vi "Begin.vi"(11 "Image Size":T3=enum."160x120") -> (0 "error out":errorcluster)   [LabVIEW 2011]
doc: "Called before other user functions, this VI is expected to open initial I/O refnums, load in file data, and do all program initialization. Notice that the <B>error out</B> terminal is simply used for data flow. Wiring it to other structures or subVIs ensures that this VI runs first."
uses:
  <vilib>/Rock Robotics/WPI/Camera/WPI_CameraImageSize.ctl
  <vilib>/Rock Robotics/SystemInterfaces/AI/FPGA_AIGyroChannel.ctl
  <vilib>/Rock Robotics/SystemInterfaces/Typedef/FPGA_TypedefAnalogModuleForGyro.ctl
  <vilib>/Rock Robotics/WPI/Joystick/WPI_JoystickDeviceEnum.ctl
  <vilib>/Rock Robotics/WPI/Camera/WPI_CameraWhite Balance Values.ctl
  <vilib>/Rock Robotics/WPI/Camera/WPI_CameraExposure Values.ctl
  <vilib>/Rock Robotics/WPI/Camera/WPI_CameraFrameRate.ctl
  <vilib>/Rock Robotics/WPI/CAN/Jaguar/SubVIs/WPI_CANJaguar_BrakeCoastMode.ctl
  <vilib>/Rock Robotics/WPI/CAN/Jaguar/SubVIs/WPI_CANJaguar_ControlMode.ctl
  <vilib>/Rock Robotics/SystemInterfaces/DIO/FPGA_DIORelayChannel.ctl
  <vilib>/Rock Robotics/SystemInterfaces/Typedef/FPGA_TypedefDigitalModule.ctl
  <vilib>/Rock Robotics/SystemInterfaces/DIO/FPGA_DIOPWMChannel.ctl
  <vilib>/Rock Robotics/WPI/MotorControl/WPI_MotorControlOpenCANJaguar.vi
  <vilib>/Rock Robotics/WPI/RobotDrive/WPI_RobotDriveOpen2MotorWithExistingMotors.vi
  <vilib>/Rock Robotics/WPI/MotorControl/WPI_MotorControlOpen Jaguar.vi
panel:
  in  "Analog Module":T1
  in  "Gain (VoltsPerDegree/Second)":dbl=0.0125
  in  "Channel":T2=enum."AI 2"
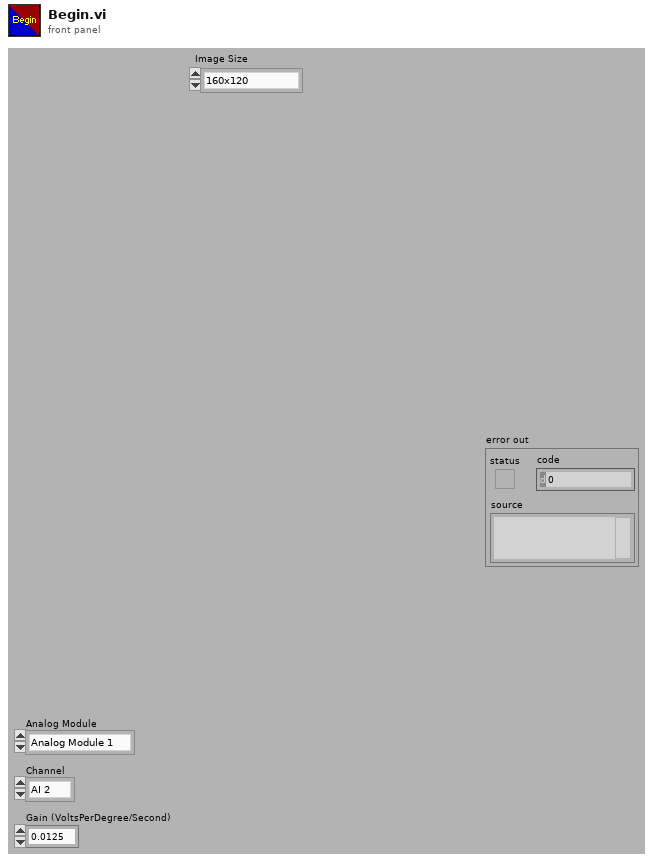
[diagram p1: front panel]
types:
  T1 = typedef "FPGA_TypedefAnalogModuleForGyro.ctl" = enum16{"Analog Module 1"}
  T2 = typedef "FPGA_AIGyroChannel.ctl" = enum8{"AI 1", "AI 2", "Invalid"}
  T3 = typedef "WPI_CameraImageSize.ctl" = enum16{"640x480", "320x240", "160x120"}
  T4 = typedef "FPGA_DIOPWMChannel.ctl" = enum8{"PWM 1", "PWM 2", "PWM 3", "PWM 4", "PWM 5", "PWM 6", "PWM 7", "PWM 8", "PWM 9", "PWM 10", "Invalid"}
  T5 = typedef "FPGA_TypedefDigitalModule.ctl" = enum16{"Digital Module 1", "Digital Module 2"}
  T6 = typedef "FPGA_DIORelayChannel.ctl" = enum8{"Relay 1", "Relay 2", "Relay 3", "Relay 4", "Relay 5", "Relay 6", "Relay 7", "Relay 8", "Invalid"}
  T7 = typedef "WPI_JoystickDeviceEnum.ctl" = enum16{"USB 1", "USB 2", "USB 3", "USB 4", "Kinect 1", "Kinect 2"}
  T8 = typedef "WPI_CANJaguar_ControlMode.ctl" = enum8{"Percent VBus", "Current", "Speed", "Position", "Voltage"}
  T9 = typedef "WPI_CANJaguar_BrakeCoastMode.ctl" = enum8{"Jumper", "Brake", "Coast"}
  T10 = typedef "WPI_CameraFrameRate.ctl" = u32
  T11 = typedef "WPI_CameraExposure Values.ctl" = enum16{"Auto", "Flicker-free 50 Hz", "Flicker-free 60 Hz", "Hold current"}
  T12 = typedef "WPI_CameraWhite Balance Values.ctl" = enum16{"Auto", "Fixed indoor", "Fixed outdoor 1", "Fixed outdoor 2", "Fixed fluorescent 1", "Fixed fluorescent 2", "Hold current"}
  T13 = typedef "WPI_JoystickDevRef.ctl" = cluster{"Device":T7}
  T14 = typedef "WPI_GyroDevRef.ctl" = cluster{"DevStatus":errorcluster, "Analog Module":T15, "Analog Channel":T16, "Offset":dbl, "Gain (VoltsPerDegree/Second)":dbl}
  T15 = typedef "FPGA_TypedefAnalogModule.ctl" = enum16{"Analog Module 1", "Analog Module 2"}
  T16 = typedef "FPGA_AIChannel.ctl" = enum8{"AI 1", "AI 2", "AI 3", "AI 4", "AI 5", "AI 6", "AI 7", "AI 8", "Invalid"}
  T17 = typedef "WPI_MotorControlDeviceRef.ctl" = cluster{"DeviceStatus":errorcluster, "Type":enum16{"PWM", "CAN"}, "PWM":cluster{"Digital Module":T5, "PWM Channel":T4, "DeadBand":T18}, "CAN":cluster{"Device Number":u8, "Control Mode":T8, "Semaphore":T19, "Max Vout":dbl}, "Invert":bool, "TransformRef":T20, "InvTransformRef":T20}
  T18 = typedef "WPI_PWMDeadband.ctl" = cluster{"Name":string, "maxPositivePwm":i32, "minPositivePwm":i32, "centerPwm":i32, "maxNegativePwm":i32, "minNegativePwm":i32, "angularRange":u16}
  T19 = typedef "Semaphore RefNum" = refnum<k1>
  T20 = typedef "WPI_PWMTransform_ConPane.ctl" = refnum<vi>
  T21 = typedef "WPI_RelayDevRef.ctl" = cluster{"DevStatus":errorcluster, "Relay Channel":T6, "Digital Module":T5, "Relay Direction":T22}
  T22 = typedef "WPI_RelayDirection.ctl" = enum16{"Both directions", "Forward only", "Reverse only"}
  T23 = typedef "WPI_CameraDevRef.ctl" = cluster{"Camera Address":string, "CameraStatus":errorcluster, "Acquire Image Notifier":refnum<notifier>}
  T24 = typedef "WPI_RobotDriveDevRef.ctl" = cluster{"DevStatus":errorcluster, "Motors[]":T17[], "Square Inputs":bool, "Max Output":dbl, "Isochronous":bool}
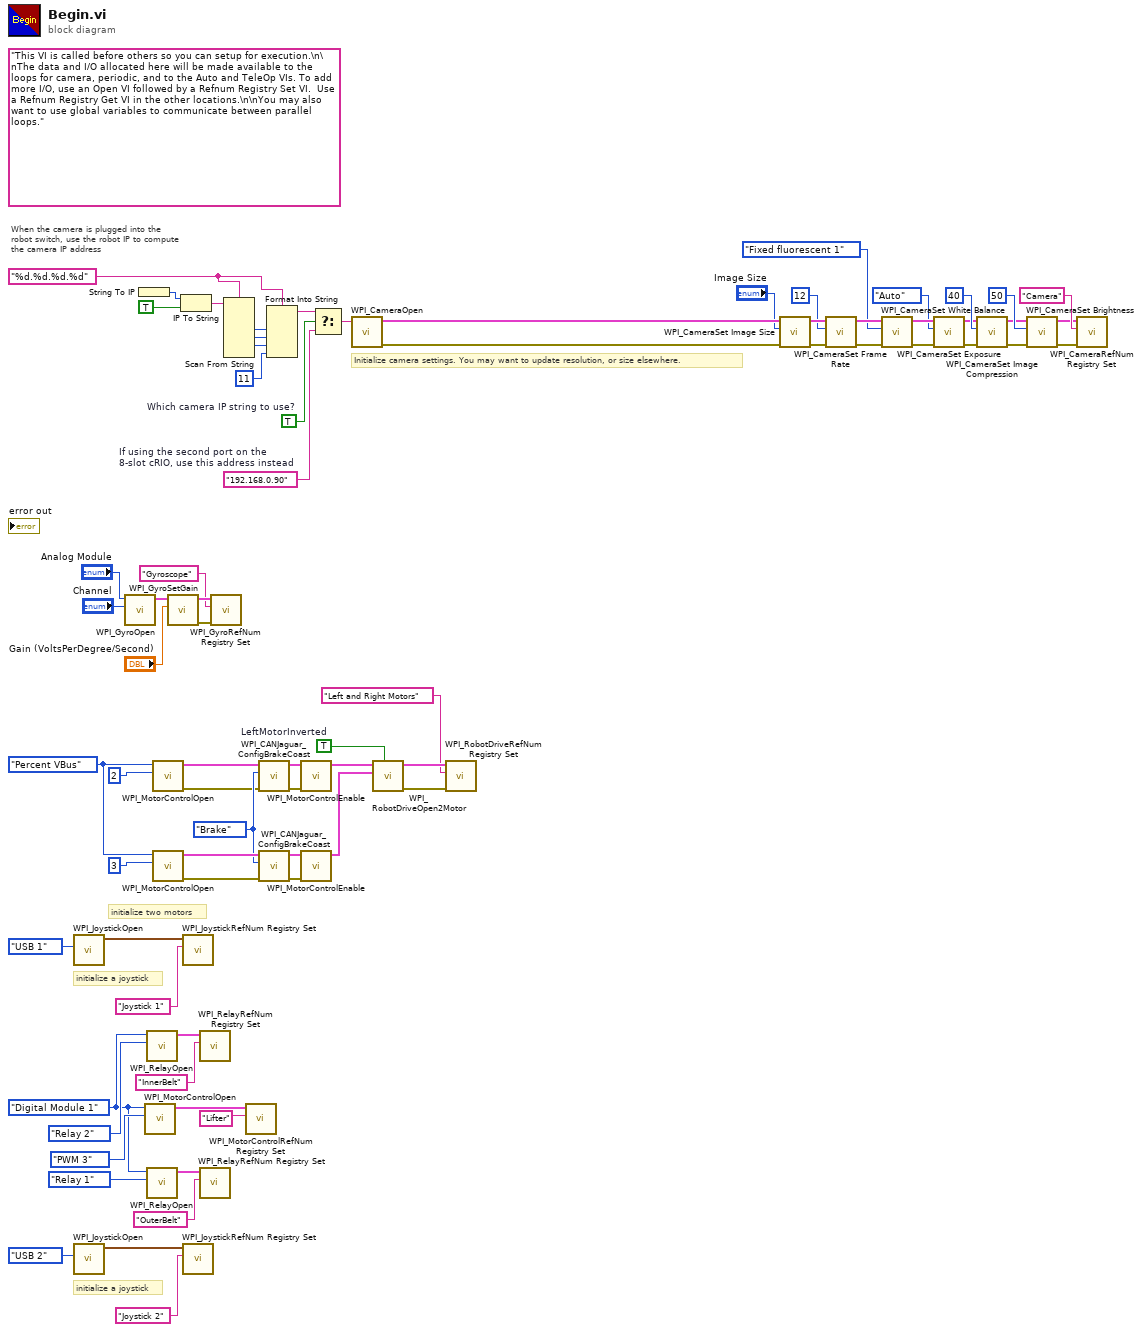
[diagram p0: block diagram]
diagram:
  w1 = FPGA_TypedefDigitalModule."Digital Module 1" ("Digital Module (Module 1)")
  w22 = WPI_CANJaguar_ControlMode."Percent VBus" ("Control Mode")
  w23 = WPI_CANJaguar_BrakeCoastMode."Brake" ("Brake / Coast Mode")
  w35 = TRUE  # Which camera IP string to use?
  w39 = "%d.%d.%d.%d" ("format string")
  (unwired) "This VI is called before others so you can setup for execution.\n\nThe data and I/O allocated here will be made available to the loops for camera, periodic, and to the Auto and TeleOp VIs. To add more I/O, use an Open VI followed by a Refnum Registry Set VI.  Use a Refnum Registry Get VI in the other locations.\n\nYou may also want to use global variables to communicate between parallel loops."
  w36 = "192.168.0.90"  # If using the second port on the 8-slot cRIO, use this address instead
  w74 = TRUE  # LeftMotorInverted
  # "initialize a joystick"
  # "When the camera is plugged into the\nrobot switch, use the robot IP to compute\nthe camera IP address"
  # "initialize a joystick"
  # "initialize two motors"
  # "Initialize camera settings. You may want to update resolution, or size elsewhere."
  n1 = call <vilib>:"WPI_JoystickOpen.vi"("JoystickDevice"=WPI_JoystickDeviceEnum."USB 1") -> ("JoystickDevRef"=w70:T13)  [unwired: 10 out]
  n2 = call <vilib>:"WPI_JoystickOpen.vi"("JoystickDevice"=WPI_JoystickDeviceEnum."USB 2") -> ("JoystickDevRef"=w13:T13)  [unwired: 10 out]
  n3 = call <vilib>:"WPI_GyroOpen.vi"("Analog Channel"="Channel", "Analog Module (Module 1)"="Analog Module") -> ("GyroDevRef"=w33:T14)  [unwired: 4 in, 5 out]
  n4 = String To IP() -> (0:w46:u32)  [unwired: 1 in]
  n5 = call-poly <vilib>:"WPI_MotorControlOpen.vi"("PWM Channel"=FPGA_DIOPWMChannel."PWM 3", "Digital Module (Module 1)"=w1) -> ("MotorControlDeviceRef"=w4:T17)  [unwired: 8 in, 1 out]
  n6 = call <vilib>:"WPI_RelayOpen.vi"("Relay Channel"=FPGA_DIORelayChannel."Relay 2", "Digital Module (Module 1)"=w1) -> ("RelayDevRef"=w8:T21)  [unwired: 8 in, 1 out]
  n7 = call <vilib>:"WPI_RelayOpen.vi"("Relay Channel"=FPGA_DIORelayChannel."Relay 1", "Digital Module (Module 1)"=w1) -> ("RelayDevRef"=w10:T21)  [unwired: 8 in, 1 out]
  n8 = call-poly <vilib>:"WPI_MotorControlOpen.vi"("Device Number"=u8 2, "Control Mode"=w22) -> ("error out"=w21:errorcluster, "MotorControlDeviceRef"=w27:T17)  [unwired: 8 in]
  n9 = call-poly <vilib>:"WPI_MotorControlOpen.vi"("Device Number"=u8 3, "Control Mode"=w22) -> ("error out"=w18:errorcluster, "MotorControlDeviceRef"=w25:T17)  [unwired: 8 in]
  n10 = call <vilib>:"WPI_GyroSetGain.vi"("Gain (VoltsPerDegree/Second)"="Gain (VoltsPerDegree/Second)", "GyroDevRef"=w33) -> ("error out"=w29:errorcluster, "GyroDevRef"=w30:T14)  [unwired: 1 in, 7 out]
  n11 = IP To String(1:TRUE ("dot notation? (F)"), 2:w46) -> (0:w44:string)
  n12 = call <vilib>:"WPI_JoystickRefNum Registry Set.vi"("refnum name"="Joystick 1", "JoystickDevRef"=w70) -> ()  [unwired: 1 in, 9 out]
  n13 = call <vilib>:"WPI_JoystickRefNum Registry Set.vi"("refnum name"="Joystick 2", "JoystickDevRef"=w13) -> ()  [unwired: 1 in, 9 out]
  n14 = call <vilib>:"WPI_RelayRefNum Registry Set.vi"("refnum name"="InnerBelt", "RelayDevRef"=w8) -> ()  [unwired: 8 in, 2 out]
  n15 = call <vilib>:"WPI_RelayRefNum Registry Set.vi"("refnum name"="OuterBelt", "RelayDevRef"=w10) -> ()  [unwired: 8 in, 2 out]
  n16 = call <vilib>:"WPI_GyroRefNum Registry Set.vi"("error in (no error)"=w29, "refnum name"="Gyroscope", "GyroDevRef"=w30) -> ()  [unwired: 7 in, 2 out]
  n17 = Scan From String(format string=w39, input string=w44) -> (output 1=w43:i32, output 2=w42:i32, output 3=w41:i32)  [unwired: 7 in, 3 out]
  n18 = call <vilib>:"WPI_MotorControlRefNum Registry Set.vi"("refnum name"="Lifter", "MotorControlDevRef"=w4) -> ()  [unwired: 8 in, 2 out]
  n19 = call <vilib>:"WPI_CANJaguar_ConfigBrakeCoast.vi"("error in (no error)"=w21, "Brake / Coast Mode"=w23, "CAN Jaguar Ref"=w27) -> ("error out"=w20:errorcluster, "CAN Jaguar Ref Out"=w26:T17)  [unwired: 7 in]
  n20 = call <vilib>:"WPI_CANJaguar_ConfigBrakeCoast.vi"("error in (no error)"=w18, "Brake / Coast Mode"=w23, "CAN Jaguar Ref"=w25) -> ("error out"=w19:errorcluster, "CAN Jaguar Ref Out"=w24:T17)  [unwired: 7 in]
  n21 = Format Into String(format string=w39, w43, w42, w41, 11 ("Compression")) -> (resulting string=w37:string)  [unwired: 2 in, 1 out]
  n22 = call <vilib>:"WPI_MotorControlEnable.vi"("error in (no error)"=w20, "CAN Jaguar Ref"=w26) -> ("CAN Jaguar Ref Out"=w16:T17)  [unwired: 8 in, 1 out]
  n23 = call <vilib>:"WPI_MotorControlEnable.vi"("error in (no error)"=w19, "CAN Jaguar Ref"=w24) -> ("CAN Jaguar Ref Out"=w17:T17)  [unwired: 8 in, 1 out]
  n24 = Select(t=w37, s=w35, f=w36) -> (s? t:f=w38:string)
  n25 = call <vilib>:"WPI_CameraOpen.vi"("Camera Address"=w38) -> ("error out"=w59:errorcluster, "CameraDevRef"=w60:T23)  [unwired: 1 in, 8 out]
  n26 = call-poly <vilib>:"WPI_RobotDriveOpen2Motor.vi"("Square Inputs"=w74, "Right Motor Dev Ref"=w17, "Left Motor Dev Ref"=w16) -> ("error out"=w68:errorcluster, "RobotDriveDevRef"=w72:T24)  [unwired: 2 in, 5 out]
  n27 = call <vilib>:"WPI_RobotDriveRefNum Registry Set.vi"("error in (no error)"=w68, "refnum name"="Left and Right Motors", "RobotDriveDevRef"=w72) -> ()  [unwired: 9 out]
  n28 = call <vilib>:"WPI_CameraSet Image Size.vi"("error in (no error)"=w59, "Image Size"="Image Size", "CameraDevRef"=w60) -> ("error out"=w58:errorcluster, "CameraDevRef Out"=w61:T23)  [unwired: 7 out]
  n29 = call <vilib>:"WPI_CameraSet Frame Rate.vi"("error in (no error)"=w58, "Frame Rate (fps)"=T10 12, "CameraDevRef"=w61) -> ("error out"=w57:errorcluster, "CameraDevRef Out"=w63:T23)  [unwired: 7 out]
  n30 = call <vilib>:"WPI_CameraSet White Balance.vi"("error in (no error)"=w57, "White Balance"=WPI_CameraWhite_Balance_Values."Fixed fluorescent 1", "CameraDevRef"=w63) -> ("error out"=w56:errorcluster, "CameraDevRef Out"=w62:T23)  [unwired: 7 out]
  n31 = call <vilib>:"WPI_CameraSet Exposure.vi"("error in (no error)"=w56, "Exposure"=WPI_CameraExposure_Values."Auto", "CameraDevRef"=w62) -> ("error out"=w55:errorcluster, "CameraDevRef Out"=w65:T23)  [unwired: 7 out]
  n32 = call <vilib>:"WPI_CameraSet Image Compression.vi"("error in (no error)"=w55, "Compression"=40, "CameraDevRef"=w65) -> ("error out"=w54:errorcluster, "CameraDevRef Out"=w64:T23)  [unwired: 7 out]
  n33 = call <vilib>:"WPI_CameraSet Brightness.vi"("error in (no error)"=w54, "Brightness"=50, "CameraDevRef"=w64) -> ("error out"=w52:errorcluster, "CameraDevRef Out"=w53:T23)  [unwired: 7 out]
  n34 = call <vilib>:"WPI_CameraRefNum Registry Set.vi"("error in (no error)"=w52, "refnum name"="Camera", "CameraDevRef"=w53) -> ()  [unwired: 9 out]
